vi "NewControl260354259.vi"(8 "error in (no error)":errorcluster, 9 "asdf":dbl, 10 "String":string, 11 "module in":refnum<class "TemplateModule.lvclass">) -> (0 "error out":errorcluster, 3 "module out":refnum<class "TemplateModule.lvclass">)   [LabVIEW 2024]
uses:
  TemplateModule.lvclass/TemplateModule.ctl
  JQMHCore/Module/RQMHModule.lvclass
  NewControl260354259.ctl
  TemplateModule.lvclass
  C:/Github/JQMH/JQMHCore/Module/RQMHModule.lvclass
  C:/Github/JQMH/Scripting/templates/TemplateModule/TemplateModule.lvclass
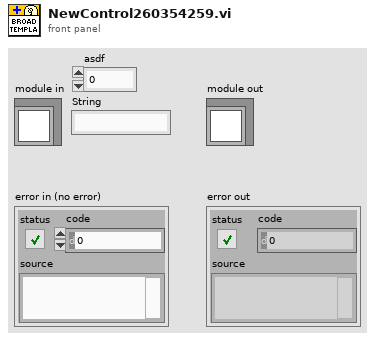
[diagram p1: front panel]
types:
  T1 = typedef "TemplateModule.lvclass/NewControl260354259.ctl" = cluster{"Module":refnum<class "RQMHModule.lvclass">, "asdf":dbl, "String":string}
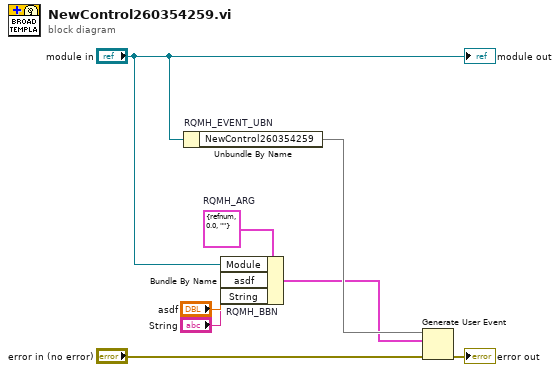
[diagram p0: block diagram]
diagram:
  w5 = T1 {"Module"=refnum, "asdf"=0.0, "String"=""}  # RQMH_ARG
  n1 = Unbundle By Name "RQMH_EVENT_UBN"("module in") -> ("NewControl260354259"=w8)
  n2 = Bundle By Name "RQMH_BBN"(cluster=w5, "Module"="module in", "asdf"="asdf", "String"="String") -> (w4:T1)
  n3 = Generate User Event(user event=w8, event data cluster=w4, error in="error in (no error)") -> (error out=→"error out":errorcluster)  [unwired: 1 in, 1 out]
  "module out" <- "module in"
